vi "ElectrodeWrite.vi"(8 "error in (no error)":errorcluster, 10 "Pulse Configuration":T1={"Charge Balance"=TRUE, "Signal Amplitude"=1, "Signal Frequency [Hz]"=160, "Signal Duration [s]"=1.0, "Delay Time [s]"=0.0, "Pulse Width [s]"=0.005} {"Pulse Width [s]" format="%0.2p"; "Delay Time [s]" format="%0.2p"; "Signal Amplitude" format="%0.0p"; "Signal Duration [s]" format="%0.2p"}, 11 "Electrode in":refnum<class "Electrode.lvclass">) -> (0 "error out":errorcluster, 3 "Electrode out":refnum<class "Electrode.lvclass">)   [LabVIEW 2012, in "Electrode.lvclass"]
uses:
  Electrode.lvclass
  PulseConfig.ctl
  Electrode.lvclass/Electrode.ctl
  StimulCtrls.lvlib
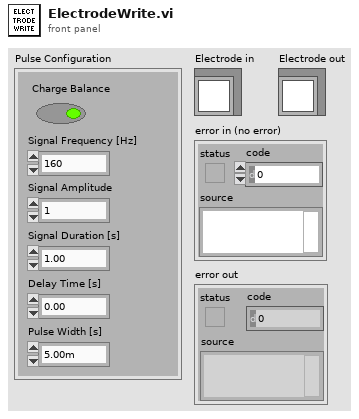
[diagram p1: front panel]
types:
  T1 = typedef "StimulCtrls.lvlib/PulseConfig.ctl" = cluster{"Charge Balance":bool, "Signal Amplitude":u32, "Signal Frequency [Hz]":u8, "Signal Duration [s]":sgl, "Delay Time [s]":sgl, "Pulse Width [s]":sgl}
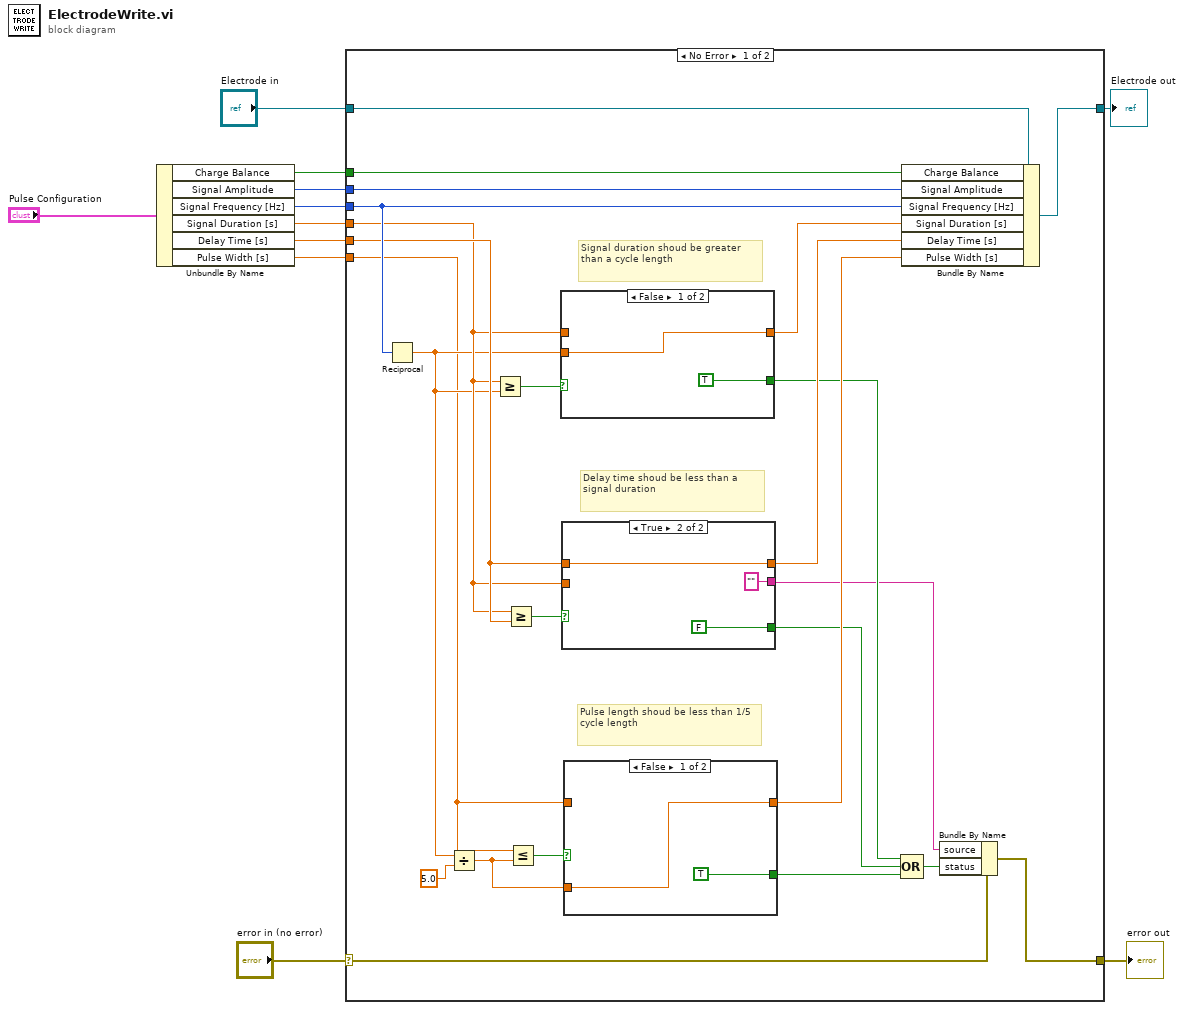
[diagram p0: block diagram]
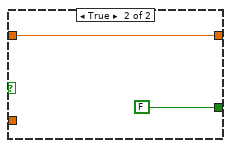
[diagram p2: hidden frame]
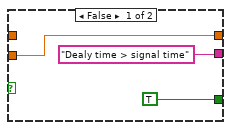
[diagram p3: hidden frame]
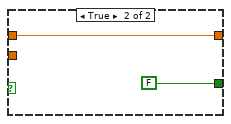
[diagram p4: hidden frame]
diagram:
  n1 = Unbundle By Name("Pulse Configuration") -> ("Charge Balance"=w6:bool, "Signal Amplitude"=w5:u32, "Signal Frequency [Hz]"=w4:u8, "Signal Duration [s]"=w3:sgl, "Delay Time [s]"=w2:sgl, "Pulse Width [s]"=w1:sgl)
  n2 = case shown="No Error" "error in (no error)" {
    selector: "error in (no error)" -> [w18 w51]
    tunnel: [w17 w51] -> w10
    tunnel: [w34 w50] -> w8
    tunnel: "Electrode in" -> [w35 w50]
    tunnel: w6 -> [w33 _]
    tunnel: w5 -> [w32 _]
    tunnel: w4 -> [w31 _]
    tunnel: w3 -> [w24 _]
    tunnel: w2 -> [w27 _]
    tunnel: w1 -> [w20 _]
    frame No Error {
      # "Pulse length shoud be less than 1/5 cycle length"
      # "Delay time shoud be less than a signal duration"
      # "Signal duration shoud be greater than a cycle length"
      n3 = Reciprocal(x=w31) -> (1/x=w23:dbl)
      n4 = Divide(x=w23, y=5.0) -> (x/y=w22:dbl)
      n5 = Greater Or Equal?(x=w24, y=w23) -> (x >= y?=w30:bool)
      n6 = Greater Or Equal?(x=w24, y=w27) -> (x >= y?=w28:bool)
      n7 = Less Or Equal?(x=w20, y=w22) -> (x <= y?=w25:bool)
      n8 = case shown="False" w30 {
        tunnel: w24 -> [_ w49]
        tunnel: [w47 w49] -> w29
        tunnel: w23 -> [w47 _]
        tunnel: [TRUE FALSE] -> w13
        frame False {
        }
        frame True {
        }
      }
      n9 = case shown="True" w28 {
        tunnel: w27 -> [_ w45]
        tunnel: [w42 w45] -> w26
        tunnel: w24 -> [w42 _]
        tunnel: [TRUE FALSE] -> w14
        tunnel: ["Dealy time > signal time" ""] -> w12
        frame False {
        }
        frame True {
        }
      }
      n10 = case shown="False" w25 {
        tunnel: w22 -> [w37 _]
        tunnel: [w37 w39] -> w19
        tunnel: w20 -> [_ w39]
        tunnel: [TRUE FALSE] -> w15
        frame False {
        }
        frame True {
        }
      }
      n11 = Compound Arithmetic op=OR(w13, w14, w15) -> (w16:bool)
      n12 = Bundle By Name(cluster=w35, "Charge Balance"=w33, "Signal Amplitude"=w32, "Signal Frequency [Hz]"=w31, "Signal Duration [s]"=w29, "Delay Time [s]"=w26, "Pulse Width [s]"=w19) -> (w34:refnum<class "Electrode.lvclass">)
      n13 = Bundle By Name(cluster=w18, "source"=w12, "status"=w16) -> (w17:errorcluster)
    }
    frame Error {
    }
  }
  "error out" <- w10
  "Electrode out" <- w8
